vi "Execute PlayPause Button.vi"(0 "reference in":refnum<class "Client.lvclass">, 5 "Play?":bool, 11 "Error In":errorcluster) -> (4 "reference out":refnum<class "Client.lvclass">, 6 "Command":T1, 15 "Error Out":errorcluster)   [LabVIEW 2024, in "Client.lvclass"]
uses:
  Client.lvclass
  Client.lvclass/Client.ctl
  Invoker/RemoteControl_class/RemoteControl.lvclass
  Support/Command Type Def.ctl
panel:
  # "Connector Pane"
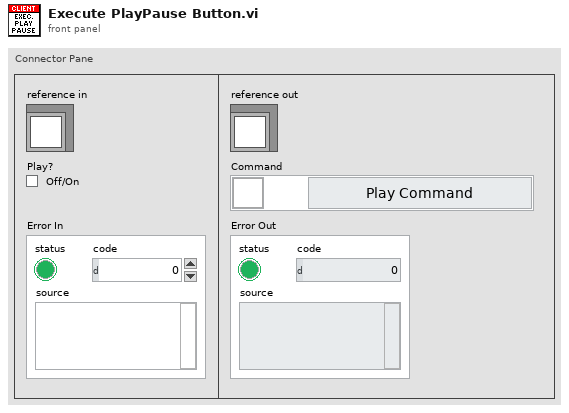
[diagram p1: front panel]
types:
  T1 = typedef "Command Type Def.ctl" = cluster{"Symbol":u16, "Command":enum16{"Play Command", "Pause Command", "Stop Command", "Rewind Command", "Skip Command", ""}}
  T2 = typedef "Client.lvclass/ObjectAttributes.ctl" = cluster{"RemoteControlRef":refnum<class "RemoteControl.lvclass">, "MediaPlayerRef":refnum<class "MediaPlayer.lvclass">, "Commands":cluster{"Play Music Command":refnum<class "IPlayerCommand.lvclass">, "Pause Music Command":refnum<class "IPlayerCommand.lvclass">, "Stop Music Command":refnum<class "IPlayerCommand.lvclass">, "Skip Music Command":refnum<class "IPlayerCommand.lvclass">, "Get Current Info Command":refnum<class "IPlayerCommand.lvclass">, "Rewind Music Command":refnum<class "IPlayerCommand.lvclass">}}
  T3 = cluster{"Play Music Command":refnum<class "IPlayerCommand.lvclass">, "Pause Music Command":refnum<class "IPlayerCommand.lvclass">, "Stop Music Command":refnum<class "IPlayerCommand.lvclass">, "Skip Music Command":refnum<class "IPlayerCommand.lvclass">, "Get Current Info Command":refnum<class "IPlayerCommand.lvclass">, "Rewind Music Command":refnum<class "IPlayerCommand.lvclass">}
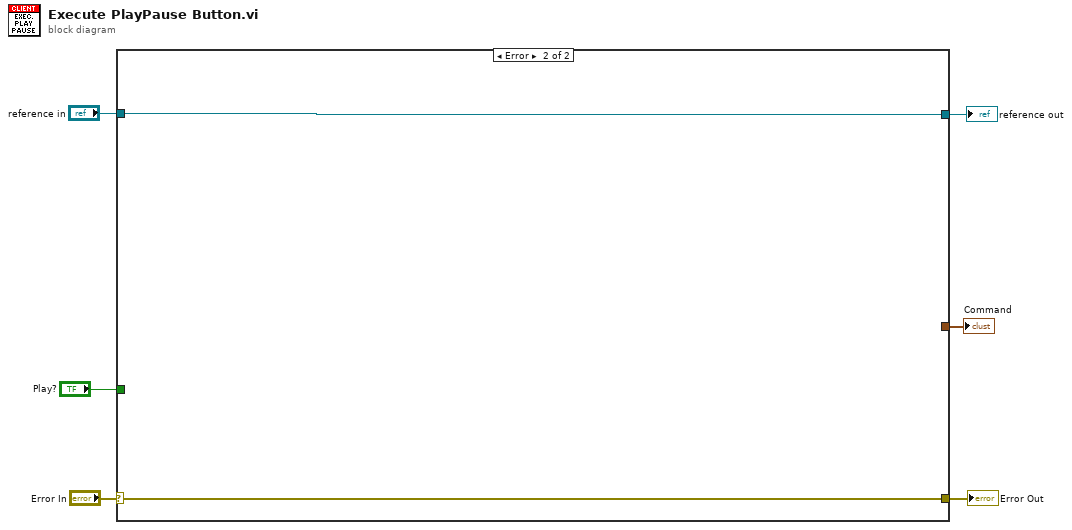
[diagram p0: block diagram]
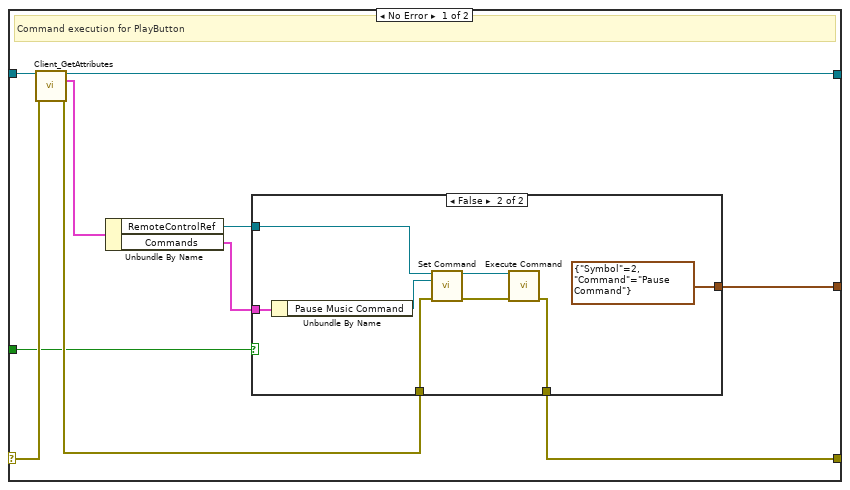
[diagram p2: hidden frame]
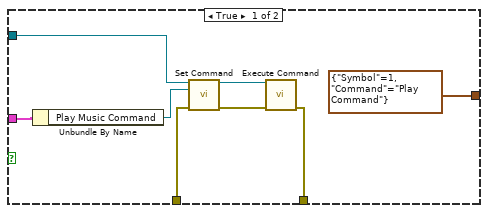
[diagram p3: hidden frame]
diagram:
  n1 = case shown="Error" "Error In" {
    selector: "Error In" -> [w16 w34]
    tunnel: [w11 w34] -> w5
    tunnel: [w12 w33] -> w3
    tunnel: "reference in" -> [w13 w33]
    tunnel: [w8 _] -> w2
    tunnel: "Play?" -> [w7 _]
    frame No Error {
      # "Command execution for PlayButton"
      n2 = call "Client_GetAttributes.vi"("reference in"=w13, "Error In"=w16) -> ("reference out"=w12:refnum<class "Client.lvclass">, "Data"=w15:T2, "Error Out"=w14:errorcluster)  [unwired: 10 in, 1 out]
      n3 = Unbundle By Name(w15) -> ("RemoteControlRef"=w10:refnum<class "RemoteControl.lvclass">, "Commands"=w9:T3)
      n4 = case shown="False" w7 {
        tunnel: w14 -> [w24 w32]
        tunnel: [w22 w30] -> w11
        tunnel: w10 -> [w20 w28]
        tunnel: w9 -> [w19 w27]
        tunnel: [T1 {"Symbol"=1, "Command"=enum."Play Command"} ("Command") T1 {"Symbol"=2, "Command"=enum."Pause Command"} ("Command")] -> w8
        frame True {
          n5 = Unbundle By Name(w19) -> ("Play Music Command"=w18:refnum<class "IPlayerCommand.lvclass">)
          n6 = call-dynamic "Set Command.vi"("reference in"=w20, "Command"=w18, "Error In"=w24) -> ("reference out"=w21:refnum<class "RemoteControl.lvclass">, "Error Out"=w23:errorcluster)  [unwired: 11 in]
          n7 = call-dynamic "Execute Command.vi"("reference in"=w21, "Error In"=w23) -> ("Error Out"=w22:errorcluster)  [unwired: 12 in, 1 out]
        }
        frame False {
          n8 = Unbundle By Name(w27) -> ("Pause Music Command"=w26:refnum<class "IPlayerCommand.lvclass">)
          n9 = call-dynamic "Set Command.vi"("reference in"=w28, "Command"=w26, "Error In"=w32) -> ("reference out"=w29:refnum<class "RemoteControl.lvclass">, "Error Out"=w31:errorcluster)  [unwired: 11 in]
          n10 = call-dynamic "Execute Command.vi"("reference in"=w29, "Error In"=w31) -> ("Error Out"=w30:errorcluster)  [unwired: 12 in, 1 out]
        }
      }
    }
    frame Error {
    }
  }
  "Error Out" <- w5
  "reference out" <- w3
  "Command" <- w2
